vi "q5 sum between p q while loop.vi"() -> ()   [LabVIEW 2025]
panel:
  out "SUM":dbl
  in  "Q":dbl
  in  "P":dbl
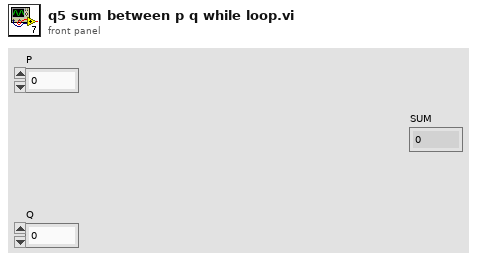
[diagram p1: front panel]
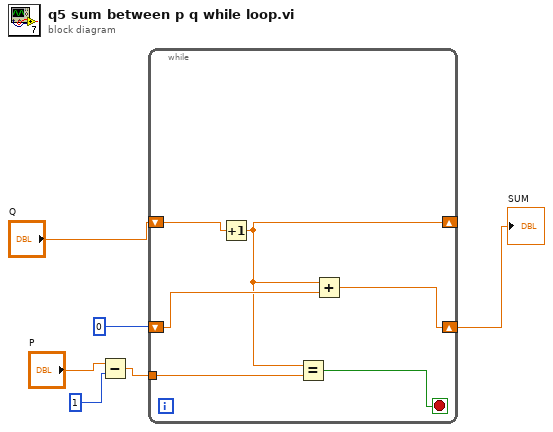
[diagram p0: block diagram]
diagram:
  n1 = Subtract(x="P", y=1) -> (x-y=w2:dbl)
  n2 = while {
    shift-right: [w9] -> _
    shift-left: "Q" -> [w12]
    shift-right: [w11] -> w1
    shift-left: 0 -> [w10]
    tunnel: w2 -> [w8]
    stop <- w7 stop-if-true
    n3 = Increment(x=w12) -> (x+1=w9:dbl)
    n4 = Equal?(x=w9, y=w8) -> (x = y?=w7:bool)
    n5 = Add(x=w9, y=w10) -> (x+y=w11:dbl)
  }
  "SUM" <- w1
